vi "Detach from Thread Network.vi"(8 "error in (no error)":errorcluster, 11 "Rocom Tests in":refnum<class "Rocom Tests.lvclass">) -> (0 "error out":errorcluster, 3 "Rocom Tests out":refnum<class "Rocom Tests.lvclass">)   [LabVIEW 2015, in "Rocom Tests.lvclass"]
uses:
  Rocom Tests.lvclass
  Classes/Manufacturing Test/Class/SC Manufacturing Test.lvclass
  <vilib>/Cree, Inc/Cree Test Framework/Classes/Base Objects/Base Class/Base Class/Base Class.lvclass
  Classes/Application/Class/Application.lvclass
  Classes/Test Recipe/Class/Test Recipe.lvclass
  Test Class/Test Class.lvclass
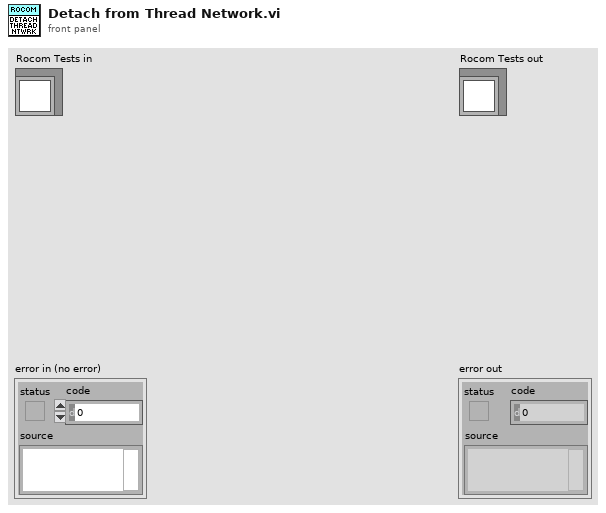
[diagram p1: front panel]
types:
  T1 = typedef "Application.lvlib/App Properties.lvclass/Class Properties -- Cluster.ctl" = cluster{"UUT Info":T2[], "Test Information":refnum<vi>, "Test Complete Event":refnum<user-event>, "Shop Floor System":refnum<class "Shop Floor System.lvclass">, "Gold Board":refnum<class "Golden Board.lvclass">, "Test Recipe":refnum<class "Test Recipe.lvclass">, "Instruments":refnum<class "Instrument.lvclass">[], "Mode":T3, "Test Results":cluster{"Pass":bool[], "Fail Codes":string[]}, "Station Config":refnum<class "Station Config.lvclass">}
  T2 = typedef "Application.lvlib/App Properties.lvclass/UUT Reference -- Cluster.ctl" = cluster{"Serial Number Reference":refnum<vi>, "Status Message Reference":refnum<vi>}
  T3 = typedef "Application.lvlib/Application.lvclass/Op Mode -- Enum.ctl" = u16
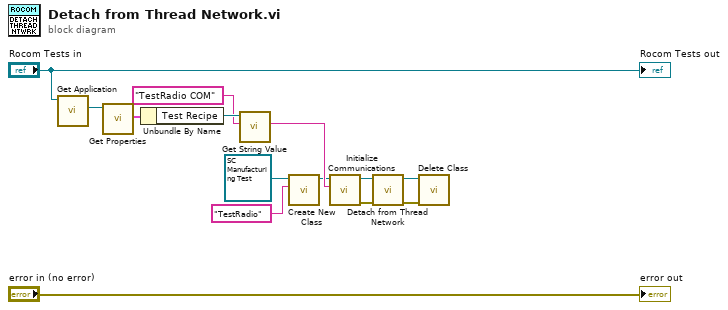
[diagram p0: block diagram]
diagram:
  n1 = call "Get Application.vi"("Test Class in"="Rocom Tests in") -> ("Application.lvlib:Application.lvclass"=w5:refnum<class "Application.lvclass">)  [unwired: 9 in, 1 out]
  n2 = call "Get Properties.vi"("Acrobat Template in"=w5) -> ("Class Properties"=w11:T1)  [unwired: 8 in, 2 out]
  n3 = Unbundle By Name(w11) -> ("Test Recipe"=w12:refnum<class "Test Recipe.lvclass">)
  n4 = call "Get String Value.vi"("Name"="TestRadio COM", "Test Recipe in"=w12) -> ("Value"=w13:string)  [unwired: 7 in, 2 out]
  n5 = call <vilib>:"Create New Class.vi"("Name"="TestRadio", "Base Class in"=refnum<class "SC Manufacturing Test.lvclass"> refnum ("SC Manufacturing Test.lvlib:SC Manufacturing Test.lvclass")) -> ("Base Class out"=w9:refnum<class "SC Manufacturing Test.lvclass">)  [unwired: 8 in, 1 out]
  n6 = call "Initialize Communications.vi"("COM Port"=w13, "Acrobat Template in"=w9) -> ("error out"=w3:errorcluster, "Acrobat Template out"=w4:refnum<class "SC Manufacturing Test.lvclass">)  [unwired: 8 in]
  n7 = call "Detach from Thread Network.vi"("error in (no error)"=w3, "Acrobat Template in"=w4) -> ("error out"=w1:errorcluster, "Acrobat Template out"=w2:refnum<class "SC Manufacturing Test.lvclass">)  [unwired: 8 in]
  n8 = call <vilib>:"Delete Class.vi"("error in (no error)"=w1, "Base Class in"=w2) -> ()  [unwired: 8 in, 2 out]
  "error out" <- "error in (no error)"
  "Rocom Tests out" <- "Rocom Tests in"
